vi "VNA Convert Frequency from MHz.vi"(10 "Units":string(combo), 11 "Frequency":dbl) -> (3 "Converted Frequency":dbl)   [LabVIEW 2011]
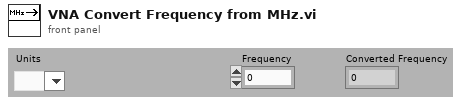
[diagram p1: front panel]
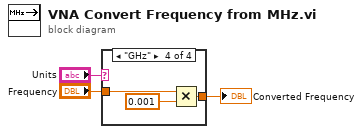
[diagram p0: block diagram]
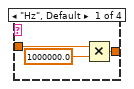
[diagram p2: hidden frame]
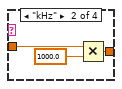
[diagram p3: hidden frame]
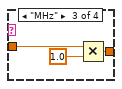
[diagram p4: hidden frame]
diagram:
  n1 = case shown="\"GHz\"" "Units" {
    tunnel: "Frequency" -> [w6 w9 w12 w15]
    tunnel: [w5 w8 w11 w14] -> w3
    frame "Hz", Default {
      n2 = Multiply(x=w6, y=1000000.0) -> (x*y=w5:dbl)
    }
    frame "kHz" {
      n3 = Multiply(x=w9, y=1000.0) -> (x*y=w8:dbl)
    }
    frame "MHz" {
      n4 = Multiply(x=w12, y=1.0) -> (x*y=w11:dbl)
    }
    frame "GHz" {
      n5 = Multiply(x=w15, y=0.001) -> (x*y=w14:dbl)
    }
  }
  "Converted Frequency" <- w3
